vi "Get all Object Items (by Offset).vi"(5 "Keep Names in JSON":bool, 8 "error in (no error)":errorcluster, 10 "Offset":i32, 11 "JSON":string) -> (0 "error out":errorcluster, 1 "Item Offsets":i32[](array[numeric]), 2 "Offset past":i32 caption="Offset past Object", 3 "Item Names":string[](array[string]), 4 "Item End Offsets":i32[](array[numeric]))   [LabVIEW 2024, in "JSONtext.lvlib"]
doc: "Return all Items in the Object as an array of Offsets to the JSON Values."
uses:
  JSONtext.lvlib
  Parsing State.ctl
  Advance past Line Ending.vi
  Advance past Number.vi
  Unescape JSON string.vi
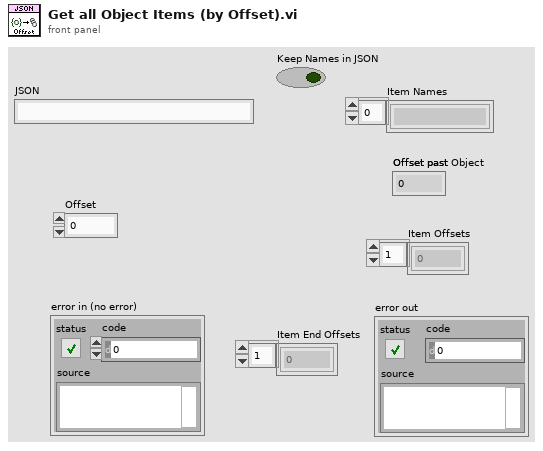
[diagram p1: front panel]
types:
  T1 = typedef "JSONtext.lvlib/Parsing State.ctl" = enum16{"Parser Error", "Object", "Array", "String", "Number/Other", "Leading Whitespace", "Object end", "Array end", "Value end"}
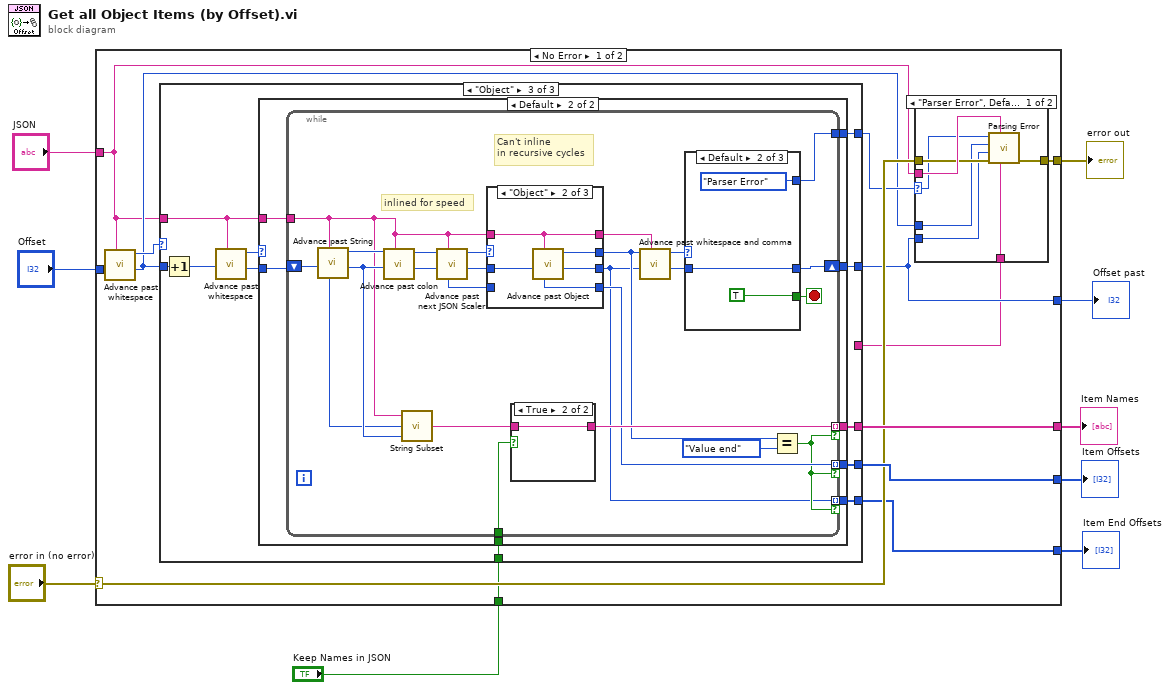
[diagram p0: block diagram]
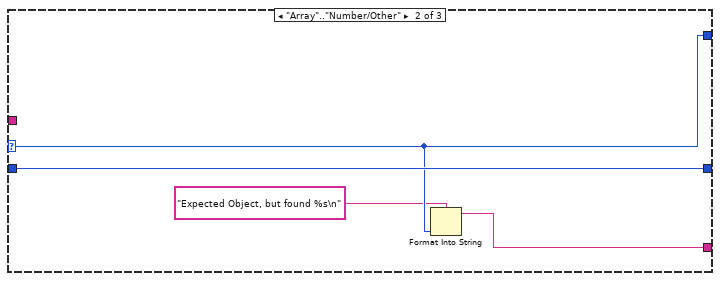
[diagram p3: hidden frame]
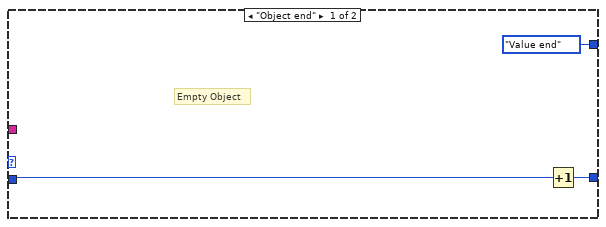
[diagram p4: hidden frame]
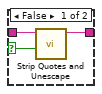
[diagram p5: hidden frame]
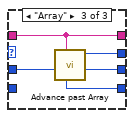
[diagram p7: hidden frame]
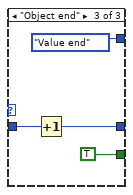
[diagram p9: hidden frame]
diagram:
  n1 = case shown="No Error" "error in (no error)" {
    selector: "error in (no error)" -> [w17 w110]
    tunnel: [w22 _] -> w9
    tunnel: [w21 _] -> w8
    tunnel: "Offset" -> [w20 w109]
    tunnel: [w18 w110] -> w6
    tunnel: [w16 w109] -> w4
    tunnel: "JSON" -> [w13 _]
    tunnel: [w11 _] -> w2
    tunnel: "Keep Names in JSON" -> [w10 _]
    frame No Error {
      n2 = call "Advance past whitespace.vi"("JSON"=w13, "Offset"=w20) -> ("Offset of first non-whitespace"=w14:i32, "Parser State"=w19:T1)  [unwired: 7 in, 1 out]
      n3 = case shown="\"Object\"" w19 {
        selector: w19 -> [w24 w26 _]
        tunnel: [w24 w26 w39] -> w15
        tunnel: [_ _ w38] -> w22
        tunnel: [_ _ w37] -> w21
        tunnel: w14 -> [w23 w28 w36]
        tunnel: w13 -> [_ _ w32]
        tunnel: [w23 w28 w35] -> w16
        tunnel: [_ w27 _] -> w12
        tunnel: [_ _ w30] -> w11
        tunnel: w10 -> [_ _ w29]
        frame "Parser Error", Default {
        }
        frame "Array".."Number/Other" {
          n4 = Format Into String(format string="Expected Object, but found %s\n", w26) -> (resulting string=w27:string)  [unwired: 2 in, 1 out]
        }
        frame "Object" {
          n5 = Increment(x=w36) -> (x+1=w34:i32)
          n6 = call "Advance past whitespace.vi"("JSON"=w32, "Offset"=w34) -> ("Offset of first non-whitespace"=w33:i32, "Parser State"=w31:T1)  [unwired: 7 in, 1 out]
          n7 = case shown="Default" w31 {
            tunnel: [Parsing_State."Value end" w50] -> w39
            tunnel: [_ w49] -> w38
            tunnel: [_ w48] -> w37
            tunnel: [w41 w47] -> w35
            tunnel: w33 -> [w40 w46]
            tunnel: w32 -> [_ w45]
            tunnel: [_ w44] -> w30
            tunnel: w29 -> [_ w43]
            frame "Object end" {
              # "Empty Object"
              n8 = Increment(x=w40) -> (x+1=w41:i32)
            }
            frame Default {
              n9 = while {
                shift-right: [w71] -> w47
                shift-left: w46 -> [w56]
                tunnel: w45 -> [w62]
                tunnel: [w69] -> w50
                tunnel: [w59] -> w49 mode=indexing if=w53
                tunnel: [w55] -> w48 mode=indexing if=w53
                tunnel: [w52] -> w44 mode=indexing if=w53
                tunnel: w43 -> [w51]
                stop <- w70 stop-if-true
                # "Can't inline\nin recursive cycles"
                # "inlined for speed"
                n10 = call "Advance past String.vi"("JSON"=w62, "Offset"=w56) -> ("Offset past match"=w63:i32, "State"=w74:T1, "Value start out"=w58:i32)  [unwired: 7 in]
                n11 = call "Advance past colon.vi"("JSON"=w62, "Offset"=w63, "State"=w74) -> ("index"=w65:i32, "State"=w66:T1)  [unwired: 7 in]
                n12 = call "String Subset.vi"("Offset past End"=w63, "Start offset"=w58, "JSON"=w62) -> ("substring"=w60:string)  [unwired: 2 in]
                n13 = call "Advance past next JSON Scaler.vi"("JSON"=w62, "Offset"=w65, "Parser State in"=w66) -> ("Offset Past"=w64:i32, "Parser State"=w67:T1, "Value start"=w57:i32)  [unwired: 6 in]
                n14 = case shown="\"Object\"" w67 {
                  selector: w67 -> [w81 _ _]
                  tunnel: w64 -> [w80 w87 w92]
                  tunnel: [w81 w86 w91] -> w54
                  tunnel: [w80 w85 w90] -> w52
                  tunnel: w62 -> [w82 w84 w89]
                  tunnel: [w82 w84 w89] -> w68
                  tunnel: [w79 w83 w88] -> w55
                  tunnel: w57 -> [w79 _ _]
                  frame Default {
                  }
                  frame "Object" {
                    n15 = call "Advance past Object.vi"("JSON"=w84, "Offset"=w87) -> ("Offset past Object"=w85:i32, "State"=w86:T1, "Object Start"=w83:i32)  [unwired: 7 in]
                  }
                  frame "Array" {
                    n16 = call "Advance past Array.vi"("JSON"=w89, "Offset"=w92) -> ("Offset past Array"=w90:i32, "State"=w91:T1, "Array Start"=w88:i32)  [unwired: 6 in, 1 out]
                  }
                }
                n17 = case shown="True" w51 {
                  selector: w51 -> [w75 _]
                  tunnel: w60 -> [w77 w78]
                  tunnel: [w76 w78] -> w59
                  frame False {
                    n18 = call "Strip Quotes and Unescape.vi"("To System Encoding (T)"=w75, "String"=w77) -> ("result string"=w76:string)  [unwired: 8 in, 1 out]
                  }
                  frame True {
                  }
                }
                n19 = call "Advance past whitespace and comma.vi"("JSON"=w68, "Offset"=w52, "State in"=w54) -> ("Offset past match"=w73:i32, "State"=w72:T1)  [unwired: 6 in, 1 out]
                n20 = case shown="Default" w72 {
                  tunnel: [_ TRUE TRUE] -> w70
                  tunnel: [_ Parsing_State."Parser Error" Parsing_State."Value end"] -> w69
                  tunnel: w73 -> [w93 w94 w98]
                  tunnel: [w93 w94 w97] -> w71
                  frame "Object".."Number/Other" {
                  }
                  frame Default {
                  }
                  frame "Object end" {
                    n21 = Increment(x=w98) -> (x+1=w97:i32)
                  }
                }
                n22 = Equal?(x=w54, y=Parsing_State."Value end") -> (x = y?=w53:bool)
              }
            }
          }
        }
      }
      n23 = case shown="\"Parser Error\", Default" w15 {
        selector: w15 -> [w102 _]
        tunnel: w13 -> [w107 _]
        tunnel: w17 -> [w106 w108]
        tunnel: [w105 w108] -> w18
        tunnel: w14 -> [w104 _]
        tunnel: w16 -> [w103 _]
        tunnel: w12 -> [w101 _]
        frame "Parser Error", Default {
          n24 = call "Parsing Error.vi"("initial string"=w101, "JSON"=w107, "error in (no error)"=w106, "Offset past match"=w103, "Value start"=w104, "State"=w102) -> ("error out"=w105:errorcluster)  [unwired: 5 in]
        }
        frame "Value end" {
        }
      }
    }
    frame Error {
    }
  }
  "Item Names" <- w9
  "Item Offsets" <- w8
  "error out" <- w6
  "Offset past" <- w4
  "Item End Offsets" <- w2
